vi "Test Logger.vi"() -> ()   [LabVIEW 2020]
panel:
  in  "Code":i32
  in  "Error Button":bool
  in  "Log Button":bool
  in  "Message":string
  in  "stop":bool
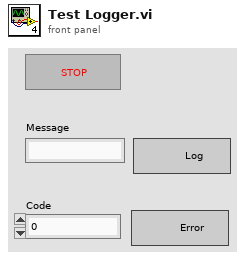
[diagram p1: front panel]
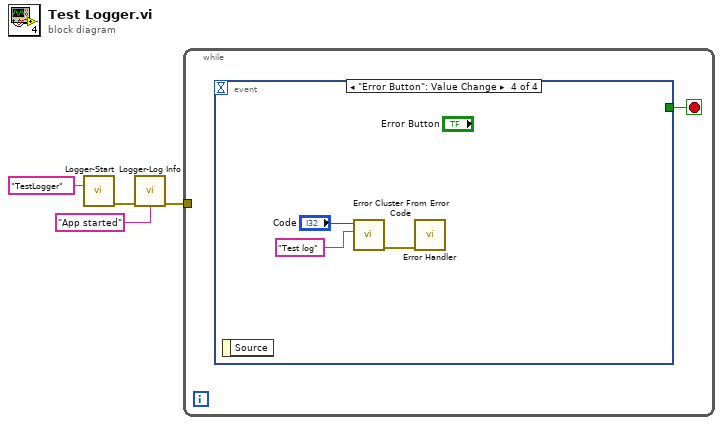
[diagram p0: block diagram]
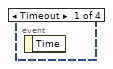
[diagram p2: hidden frame]
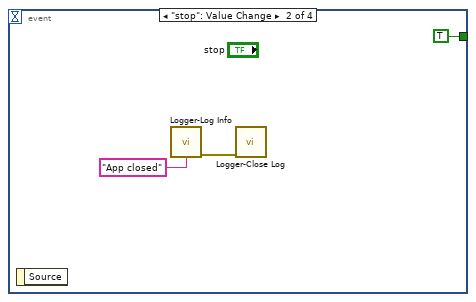
[diagram p3: hidden frame]
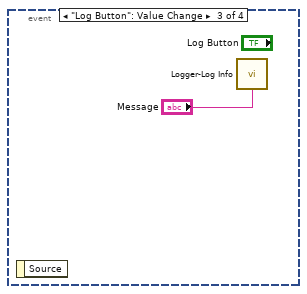
[diagram p4: hidden frame]
diagram:
  n1 = call "Logger-Start.vi"("Name"="TestLogger") -> ("error out"=w3:errorcluster)  [unwired: 14 in]
  n2 = call "Logger-Log Info.vi"("error in (no error)"=w3, "Message"="App started") -> ("error out"=w2:errorcluster)  [unwired: 13 in]
  n3 = while {
    tunnel: w2 -> [_]
    stop <- w5 stop-if-true
    n4 = event shown="[3] \"Error Button\": Value Change" {
      selector: _ -> [_ _ _ _]
      dyn-events: _ -> [_ _ _ _]
      timeout: _ -> [_ _ _ _]
      tunnel: [_ TRUE _ _] -> w5
      event Timeout {
        n5 = event-data() -> ()  [unwired: 1 in, 1 out]
      }
      event "stop": Value Change {
        n6 = event-data() -> ()  [unwired: 1 in, 1 out]
        n7 = call "Logger-Log Info.vi"("Message"="App closed") -> ("error out"=w7:errorcluster)  [unwired: 14 in]
        n8 = call "Logger-Close Log.vi"("error in (no error)"=w7) -> ()  [unwired: 14 in, 1 out]
      }
      event "Log Button": Value Change {
        n9 = event-data() -> ()  [unwired: 1 in, 1 out]
        n10 = call "Logger-Log Info.vi"("Message"="Message") -> ()  [unwired: 14 in, 1 out]
      }
      event "Error Button": Value Change {
        n11 = event-data() -> ()  [unwired: 1 in, 1 out]
        n12 = call <vilib>:"Error Cluster From Error Code.vi"("error message (\"\")"="Test log" ("error message (\"\")"), "error code (0)"="Code") -> ("error out"=w10:errorcluster)  [unwired: 7 in]
        n13 = call "Error Handler.vi"("error in (no error)"=w10) -> ()  [unwired: 12 in, 3 out]
      }
    }
  }
